vi "adri tried.vi"() -> ()   [LabVIEW 2020]
panel:
  in  "RX Slider\n\nRX Slider":dbl(slide) scale=0.0..10.0
  in  "Beam Power":dbl(slide) scale=0.0..10.0
  in  "Beam Power":dbl(slide) scale=0.0..10.0
  in  "TX Slider":dbl(slide) scale=0.0..10.0
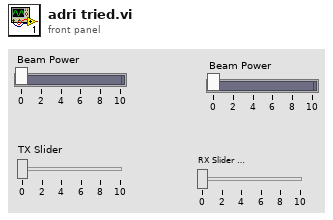
[diagram p1: front panel]
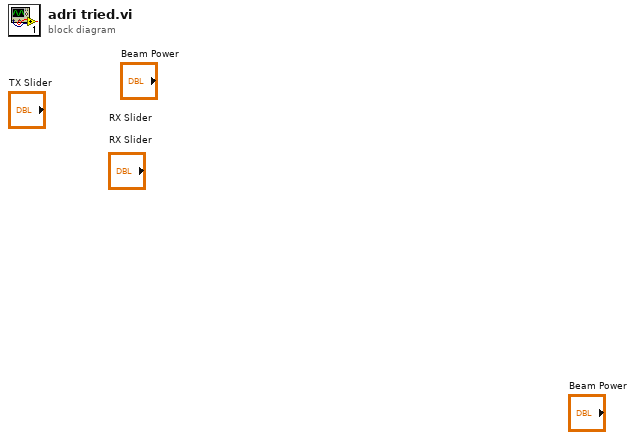
[diagram p0: block diagram]
diagram:
